vi "JSON to Package ID.vi"(11 "JSON":string) -> (3 "Package":T1)   [LabVIEW 2020, in "neg-pkg.lvlib" / "Package.lvclass"]
uses:
  Package.lvclass
  Package ID.ctl
  Package Type.ctl
  neg_pkgs/negentropicdev/lv-json/JSON/JSON.lvlib
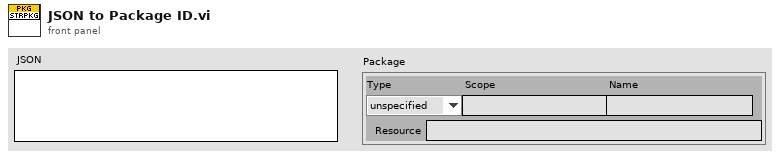
[diagram p1: front panel]
types:
  T1 = typedef "neg-pkg.lvlib/Package.lvclass/Package ID.ctl" = cluster{"Type":T2, "Scope":string, "Name":string, "Resource":string}
  T2 = typedef "neg-pkg.lvlib/Package.lvclass/Package Type.ctl" = enum16{"unspecified", "git"}
  T3 = typedef "JSON.lvlib/JSON Item Type.ctl" = enum16{"unknown", "null", "Array", "Object", "String", "Number", "Boolean"}
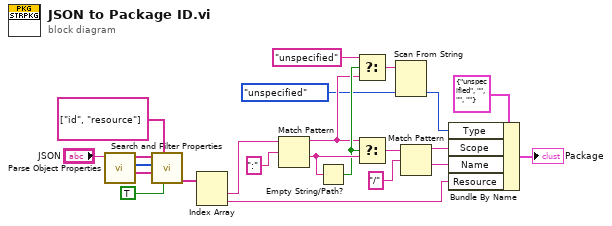
[diagram p0: block diagram]
diagram:
  n1 = call "Parse Object Properties.vi"("JSON String"="JSON") -> ("Values"=w6:string[], "Item Types"=w7:T3[], "Keys"=w8:string[])  [unwired: 7 in, 1 out]
  n2 = call "Search and Filter Properties.vi"("Remove Found? (F)"=TRUE, "Search Keys"=string[] ["id", "resource"], "Values In"=w6, "Types In"=w7, "Keys In"=w8) -> ("Filtered Values"=w1:string[])  [unwired: 1 in, 5 out]
  n3 = Index Array(array=w1) -> (element #1=w2:string, element #2=w3:string)  [unwired: 2 in]
  n4 = Match Pattern(string=w2, regular expression=":") -> (before substring=w20:string, after substring=w22:string)  [unwired: 1 in, 2 out]
  n5 = Empty String/Path?(string/path=w22) -> (empty?=w21:bool)
  n6 = Select(t="unspecified", s=w21, f=w20) -> (s? t:f=w18:string)
  n7 = Select(t=w20, s=w21, f=w22) -> (s? t:f=w16:string)
  n8 = Scan From String(input string=w18, default 1=Package_Type."unspecified" ("Package Type")) -> (output 1=w11:T2)  [unwired: 3 in, 3 out]
  n9 = Match Pattern(string=w16, regular expression="/") -> (before substring=w13:string, after substring=w12:string)  [unwired: 1 in, 2 out]
  n10 = Bundle By Name(cluster=T1 {"Type"=enum."unspecified", "Scope"="", "Name"="", "Resource"=""} ("Package"), "Type"=w11, "Scope"=w13, "Name"=w12, "Resource"=w3) -> (→"Package":T1)
